vi "Test.vi"() -> ()   [LabVIEW 2016]
panel:
  out "number":u32
  in  "3":bool=TRUE
  in  "2":bool=TRUE
  in  "1":bool=TRUE
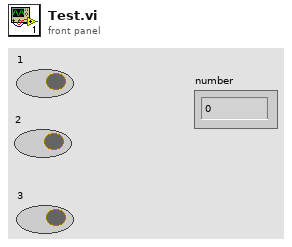
[diagram p1: front panel]
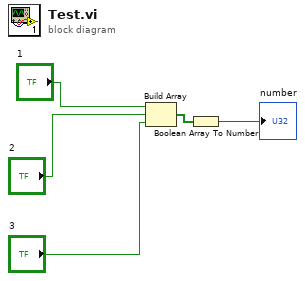
[diagram p0: block diagram]
diagram:
  n1 = Build Array("1", "2", "3") -> (w5:bool[])
  n2 = Boolean Array To Number(Boolean array=w5) -> (number=→"number":u32)
